vi "Water Control Normally Open.vi"(11 "Cooling Water Control Valve (% Closed)":dbl) -> (3 "upper limit":dbl)   [LabVIEW 2017]
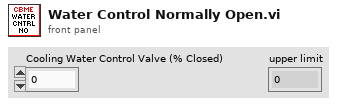
[diagram p1: front panel]
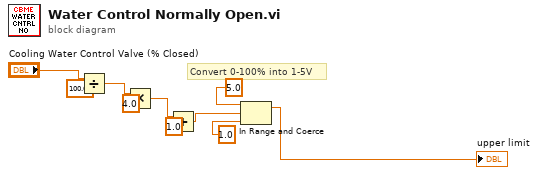
[diagram p0: block diagram]
diagram:
  # "Convert 0-100% into 1-5V"
  n1 = Divide(x="Cooling Water Control Valve (% Closed)", y=100.0) -> (x/y=w3:dbl)
  n2 = Multiply(x=w3, y=4.0) -> (x*y=w5:dbl)
  n3 = Add(x=w5, y=1.0) -> (x+y=w8:dbl)
  n4 = In Range and Coerce(upper limit=5.0, x=w8, lower limit=1.0) -> (coerced(x)=→"upper limit":dbl)  [unwired: 1 out]
